vi "Set Address Device.vi"(8 "error in (no error)":errorcluster caption="entrée d'erreur (pas d'erreur)", 10 "Address Device":refnum<visa-resource-name>, 11 "Class UART (Default) en entrée":refnum<class "Class UART (Default).lvclass">) -> (0 "error out":errorcluster caption="sortie d'erreur", 3 "Class UART (Default) en sortie":refnum<class "Class UART (Default).lvclass">)   [LabVIEW 2020, in "Library Instrument & Equipement.lvlib" / "Library UART.lvlib" / "Class UART (Default).lvclass"]
uses:
  Class UART (Default).lvclass
  Class UART (Default).lvclass/Class UART (Default).ctl
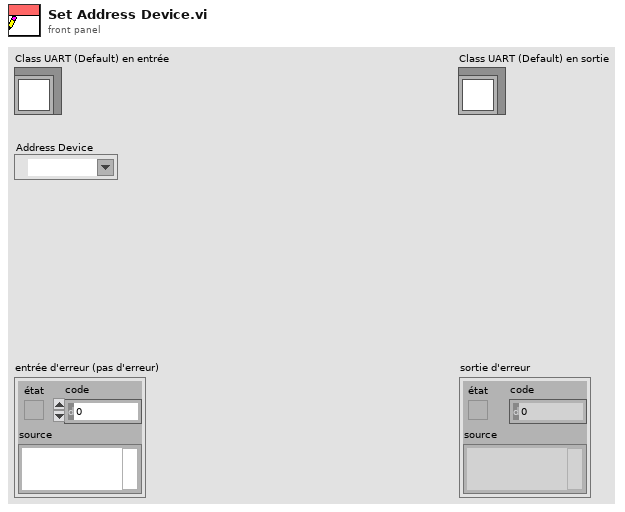
[diagram p1: front panel]
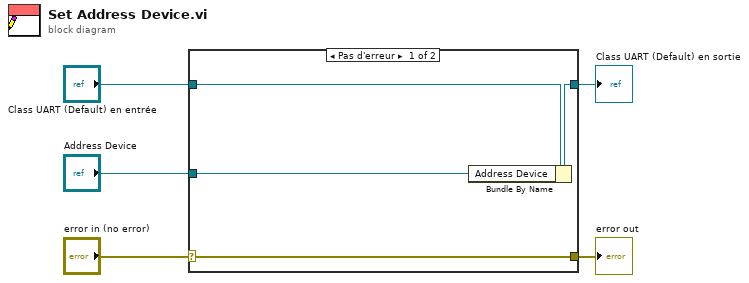
[diagram p0: block diagram]
diagram:
  n1 = case shown="Pas d'erreur" "error in (no error)" {
    selector: "error in (no error)" -> [w9 w10]
    tunnel: [w9 w10] -> w4
    tunnel: [w7 w11] -> w2
    tunnel: "Class UART (Default) en entrée" -> [w8 w11]
    tunnel: "Address Device" -> [w6 _]
    frame No Error {
      n2 = Bundle By Name(cluster=w8, "Address Device"=w6) -> (w7:refnum<class "Class UART (Default).lvclass">)
    }
    frame Error {
    }
  }
  "error out" <- w4
  "Class UART (Default) en sortie" <- w2
